vi "TagBus_Check for Tag Existance.vi"(8 "error in (no error)":errorcluster, 11 "TagBus in":refnum<class "TagBus.lvclass">) -> (0 "error out":errorcluster, 3 "TagBus out":refnum<class "TagBus.lvclass">)   [LabVIEW 2015, in "TagBus.lvclass"]
uses:
  TagBus.lvclass
  TagBus.lvclass/TagBus.ctl
  <vilib>/NI/Tag Bus/dictionary/data dictionary.lvclass
panel:
  out "Tag Not Found":bool
  in  "Controls[]":refnum<vi>[](array[refnum])
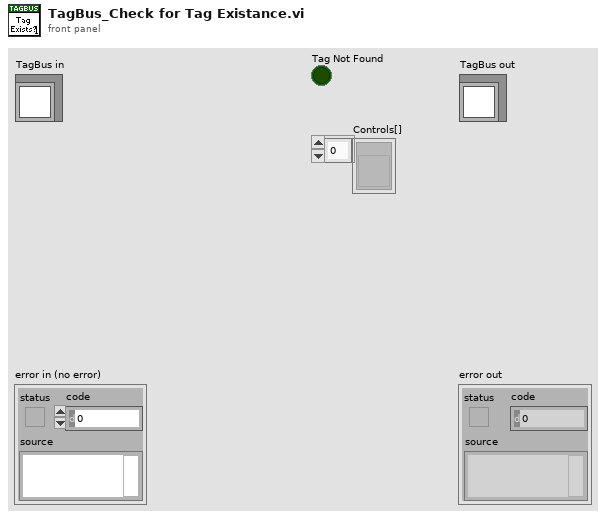
[diagram p1: front panel]
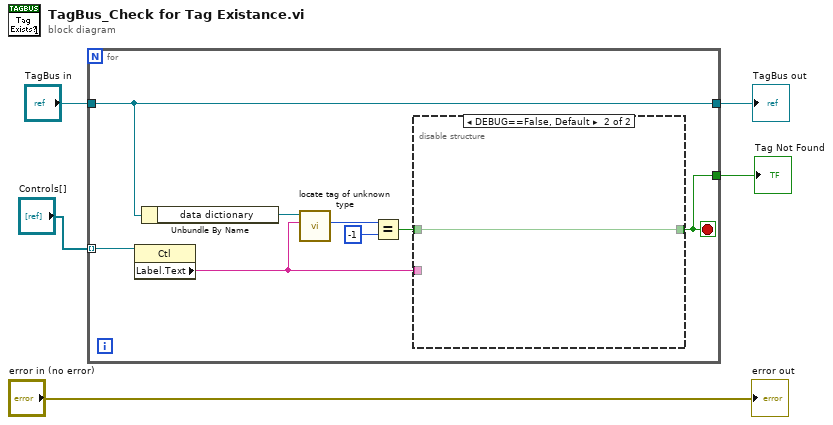
[diagram p0: block diagram]
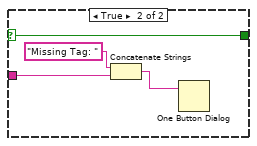
[diagram p3: hidden frame]
diagram:
  n1 = for {
    tunnel: "Controls[]" -> [w13] mode=indexing
    tunnel: "TagBus in" -> [w12]
    tunnel: [w12] -> w3
    tunnel: [w7] -> w1
    stop <- w7 stop-if-true
    n2 = property class="Ctl"(reference=w13) -> ("Label.Text"=w6:string)  [unwired: 1 in, 2 out]
    n3 = Unbundle By Name(w12) -> ("data dictionary"=w11:refnum<class "data dictionary.lvclass">)
    n4 = call <vilib>:"locate tag of unknown type.vi"("name"=w6, "data dictionary in"=w11) -> ("index"=w10:i32)  [unwired: 6 in, 3 out]
    n5 = Equal?(x=w10, y=-1) -> (x = y?=w8:bool)
    n6 = disable-structure shown="DEBUG==False, Default" {
      disable-tunnel: w8 -> [w16 w22]
      disable-tunnel: [w15 w22] -> w7
      disable-tunnel: w6 -> [w14 _]
      frame condition #0 (active) {
        n7 = case shown="False" w16 {
          selector: w16 -> [w17 w21]
          tunnel: [w17 w21] -> w15
          tunnel: w14 -> [_ w19]
          frame False {
          }
          frame True {
            n8 = Concatenate Strings("Missing Tag: ", w19) -> (w18:string)
            n9 = One Button Dialog(message=w18) -> ()  [unwired: 1 in, 1 out]
          }
        }
      }
      frame condition #1 {
      }
    }
  }
  "TagBus out" <- w3
  "Tag Not Found" <- w1
  "error out" <- "error in (no error)"
